vi "RIS.vi"(2 "Run uninterrupted?":bool, 3 "Device Category IN:":string(combo)="Short Strip" caption="Device Category:", 4 "Batch No.:":string, 5 "Wafer Serial No.:":string, 6 "Sensor Serial No.:":string) -> (0 "Done!":bool)   [LabVIEW 2013]
doc: "Performs Ris measurements according to ATLAS ITk Quality Control Specifications."
uses:
  InstrControl/SupplyControl/SupplyControl.lvclass
  general_VIs/globals/QC_RunInformation.vi
  InstrControl/ArduinoControl/ArduinoControl.lvclass
  general_VIs/globals/QC_MeasurementSetup.vi
  <vilib>/Analysis/NI_AALBase.lvlib
  InstrControl/InstrumentSetup.vi
  InstrControl/InstrControl.lvclass
  <vilib>/Analysis/6fits.llb/Curve Fitting Criteria.ctl
  <vilib>/Analysis/NI_AALPro.lvlib
  InstrControl/MultimeterControl/MultimeterControl.lvclass
  InstrControl/Switching/Switching.lvclass
panel:
  out "Ris":dbl[](array[numeric]) caption="Ris [MOhm]"
  out "Volts":dbl[](array[numeric]) caption="Volts [V]"
  out "Current":dbl[](array[numeric]) caption="Current [nA]"
  in  "No. of readouts":i32=5
  out "Risgraph":cluster{dbl[], dbl[]}(graph)
  out "Vigraph":cluster{i32[], dbl[]}[](graph)
  out "Imgraph":cluster{i32[], dbl[]}[](graph)
  out "Initial volts [V]":dbl format="%.1f"
  out "Final volts [V]":dbl=-700.0 format="%.1f"
  out "step [V]":dbl=10.0 format="%.1f"
  out "step interval [s]":u32=10
  out "Temp.":dbl[](array[numeric]) caption="Temp. [°C]" format="%#.2f"
  out "RH":dbl[](array[numeric]) caption="RH [%]" format="%#.2f"
  out "positive ramp?":bool
  out "Tab Control":enum32{"Ris Setup", "Ris Scan"}(tab)
  in  "Voltmeter":string(combo)="Keithley 2410"
  in  "Ris SMU":string(combo)="Keithley 2410"
  in  "Current \nLimit \n[µA]":dbl=1000.0 min=0.0001 format="%.3f"
  in  "Set\ncurrent\nlimit?":bool
  in  "Temperature":enum16{"Read Arduino", "Enter manually"}(ring)
  in  "Ris Supply":string(combo)="Keithley 2410"
  in  "User:":string(combo)="Christoph"
  in  "Configurations":bool
  in  "Manufacturer:":string(combo)="Hamamatsu"
  in  "Quit":bool
  in  "Continue":bool
  in  "abort":bool
  out "Device Category:":string
  out "Batch:":string
  out "Current Volts:":dbl format="%.2f"
  in  "quit (no save)":bool
  in  "Quit & Save":bool
  out "Bias On/Off:":bool
  out "STATUS 1":string
  out "Initiated:":string
  out "Sensor No.:":string
  out "No of steps":u32
  out "Current reading No.":u32
  out "Last reading at:":string
  out "Ris SMU Current [nA]":dbl[][][](array[numeric])
  out "Ris induced Voltage [V]":dbl[][][](array[numeric])
  # "University of\nCambridge"
  # "Strip Sensor QC: inter-strip Resistance"
  # "Ris Scan parameters:"
  # "Last 5 readings:"
  # "n-4"
  # "n-3"
  # "n-2"
  # "n-1"
  # "n"
  # "DUT & Test Description"
  # "Hardware"
  # "DUT & Test Description:"
  # "Current status:"
  # "Rdg No:"
  # "out of"
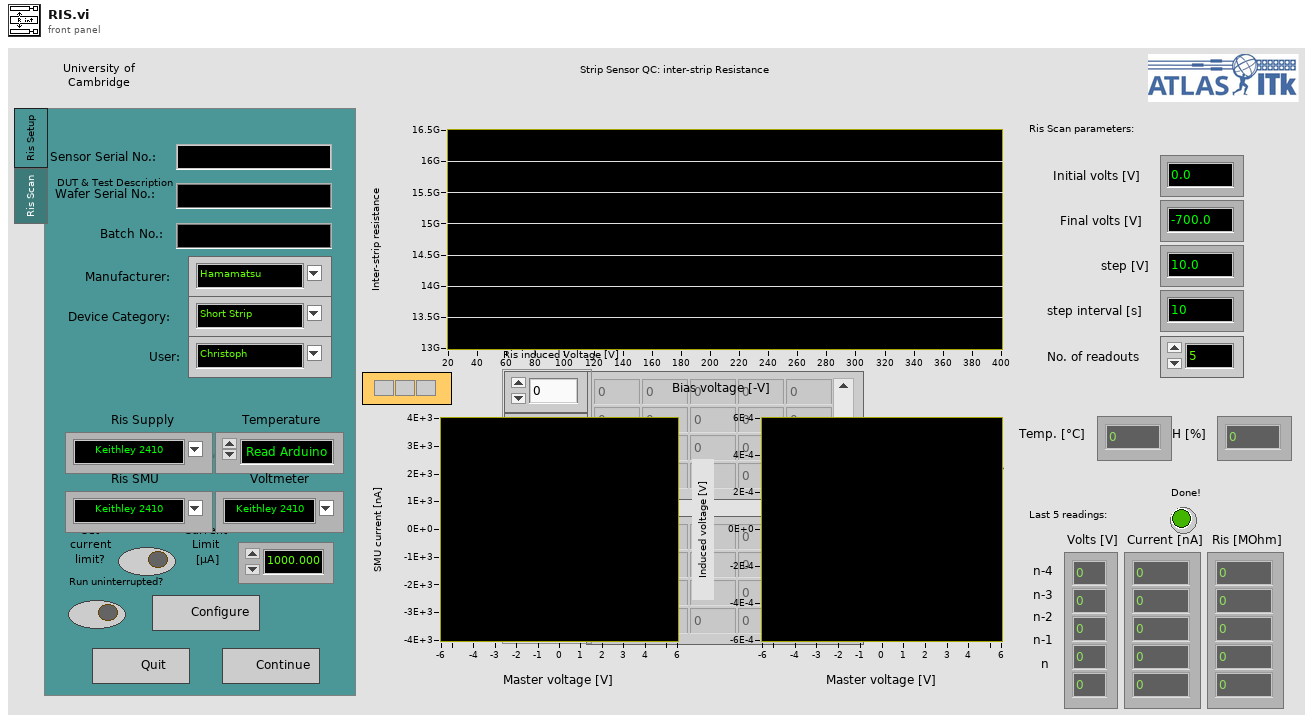
[diagram p1: front panel]
types:
  T1 = enum32{"IV", "CV", "Stability", "Striptest", "Cis", "Ris", "PTP"}
  T2 = enum16{"Supply", "LCR", "Multimeter", "Switching"}
  T3 = enum16{"Reset", "Read Array", "Read Element", "Write Element", "Write Array", "Add Element", "Add Array"}
  T4 = enum16{"Reset", "Ground", "Striptest SMU", "Striptest LCR", "IV", "CV", "Interstrip Cap", "Interstrip Res"}
  T5 = cluster{"Sensor Serial No.:":string, "Wafer:":string, "Batch:":string, "Manufacturer:":string, "Device Category:":string, "Database Serial No.:":string, "Date Initiated:":string, "Time Initiated:":string, "Test":string, "Probeplan used:":string, "End of Run comment:":string, "User:":string, "Vbias SMU":string, "LCR":string, "Test SMU":string, "Test DMM":string}
  T6 = cluster{"Institute":string, "Manufacturers":string[], "Devices":string[], "Serialnumbers Lookup DB":string, "Data directory":string, "Backup & screenshot directory":string, "List of known users":string[], "Measurement switch not used":bool, "Measurement Switch":string, "DUT Switch":string, "Rseries IV [MOhm]":string, "Rshunt IV [MOhm]":string, "Rseries CV [MOhm]":string, "DC blocking Cap [µF]":string, "Rseries LCR [MOhm]":string, "Rseries stability [MOhm]":string, "Rshunt stability [MOhm]":string, "Rseries striptest bias [MOhm]":string, "Rseries strip pinhole [MOhm]":string}
  T7 = cluster{"Bias Supply":refnum<class "SupplyControl.lvclass">, "SMU":refnum<class "SupplyControl.lvclass">, "Multimeter":refnum<class "MultimeterControl.lvclass">, "Arduino":refnum<class "ArduinoControl.lvclass">, "Measurement switch":refnum<class "Switching.lvclass">, "Initial Voltage [V]":dbl, "Final Voltage [V]":dbl, "Step Size [V]":dbl, "Step Interval [s]":i32, "Number Of Steps":u32, "Ramp down steps [V]":dbl, "Ramp down Interval [s]":i32, "Set Current Limit?":bool, "Current Limit [µA]":dbl, "Temperature Readout":enum16{"Read Arduino", "Enter manually"}, "Supply Name":string, "SMU Name":string, "Voltmeter Name":string, "R_is Limit [MOhm]":dbl, "Measurement switch used?":bool, "Matrix X Channels":cluster{"Bias Supply / SMU LO":i32, "Bias Supply / SMU HI":i32, "CV Box LO":i32, "CV Box HI":i32, "CV Box LO IN":i32, "CV Box HI IN":i32, "Volt meter LO":i32, "Volt meter HI":i32, "Mux1 C1":i32, "Mux1 C2":i32, "Mux2 C1":i32, "Mux2 C2":i32}}
  T8 = cluster{"VISA address":refnum<visa-resource-name>, "T sensor":enum16{"SHT", "DS"}, "Arduino":refnum<class "ArduinoControl.lvclass">}
  T9 = typedef "NI_AALPro.lvlib/Curve Fitting Criteria.ctl" = u16
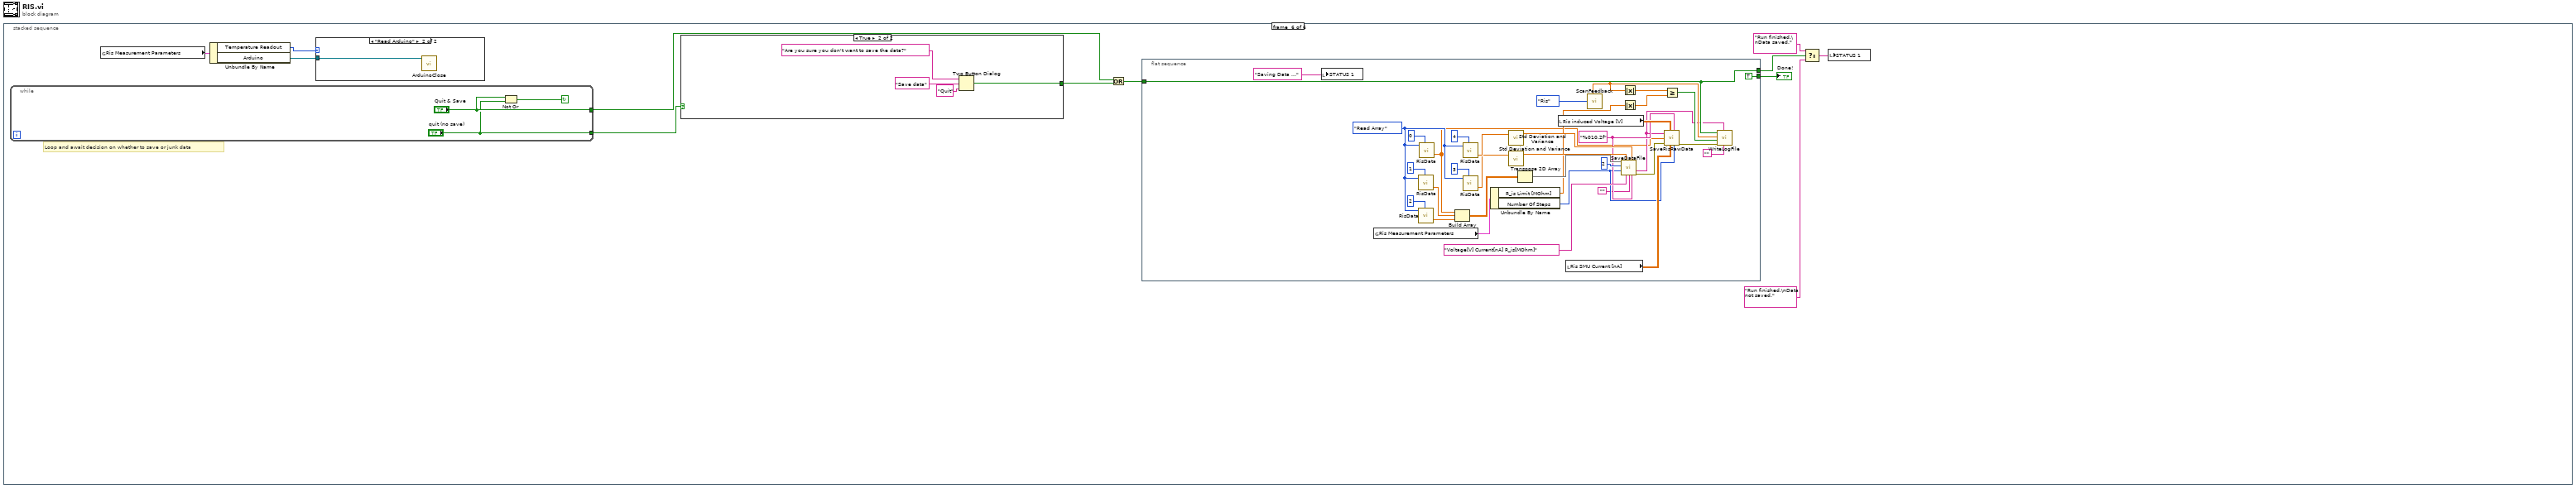
[diagram p0: block diagram]
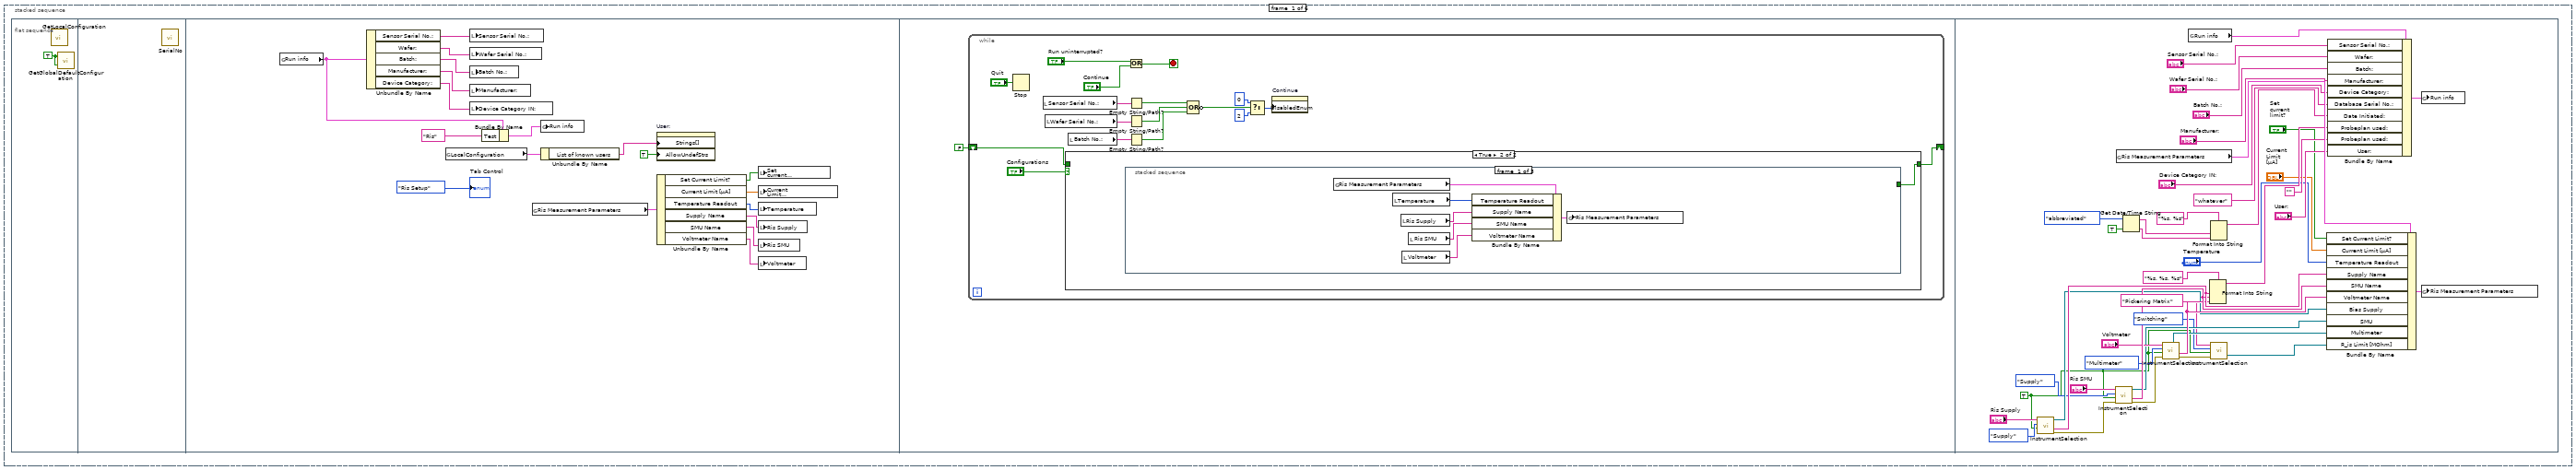
[diagram p2: hidden frame]
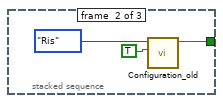
[diagram p4: hidden frame]
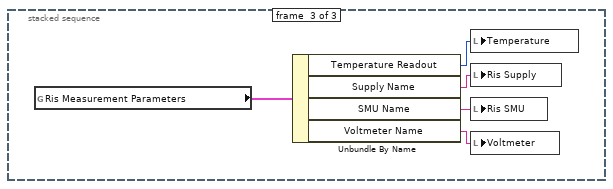
[diagram p5: hidden frame]
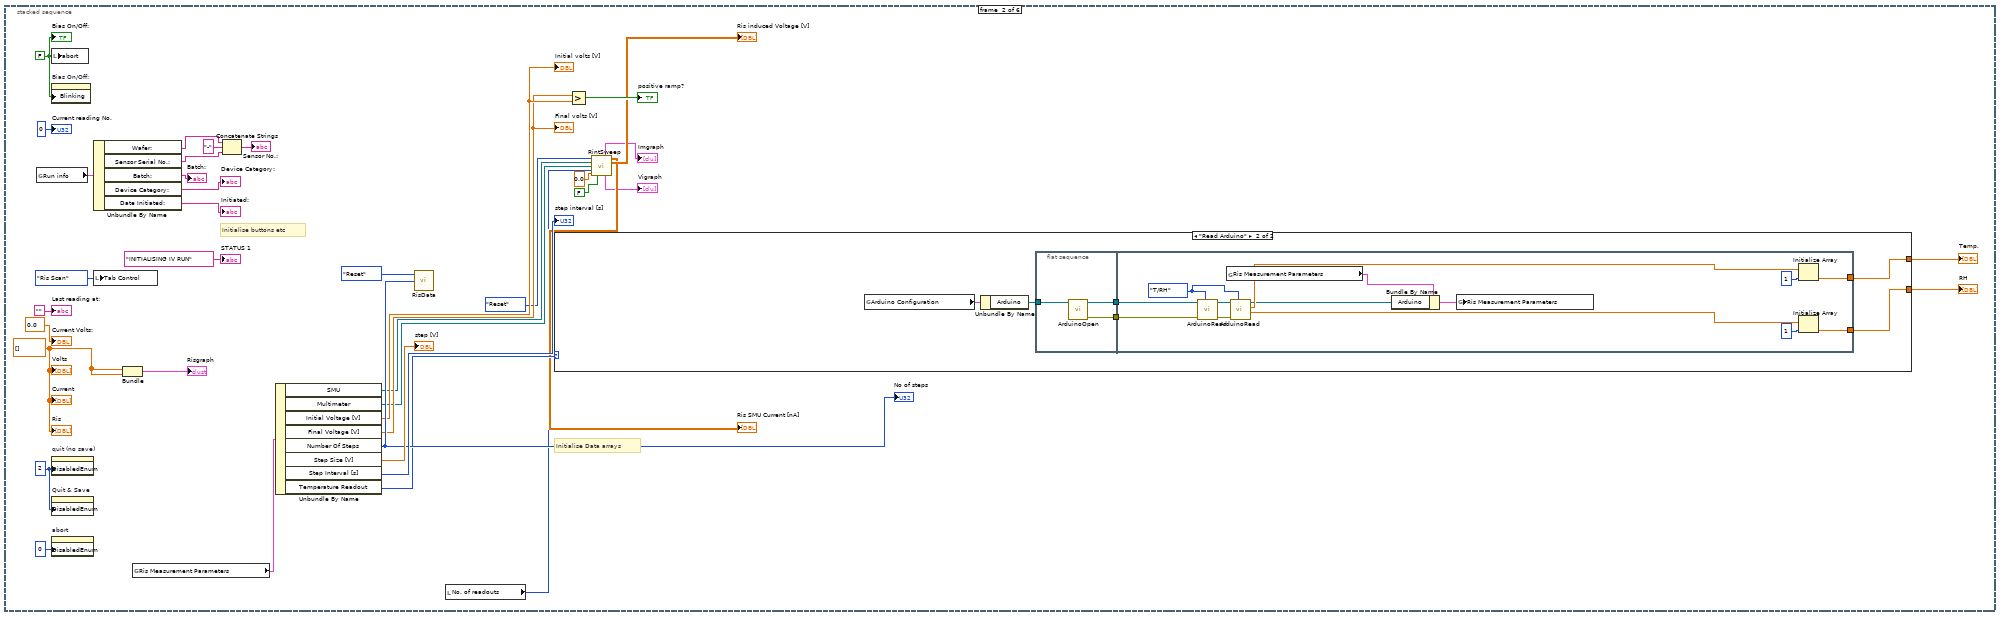
[diagram p6: hidden frame]
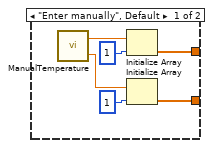
[diagram p7: hidden frame]
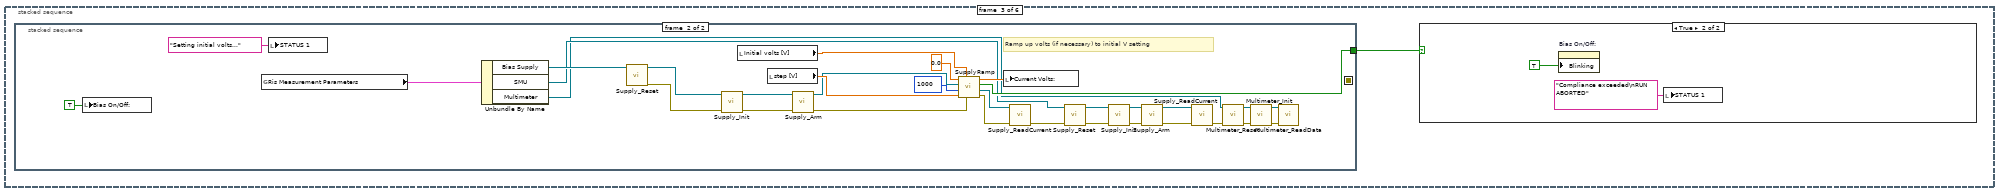
[diagram p8: hidden frame]
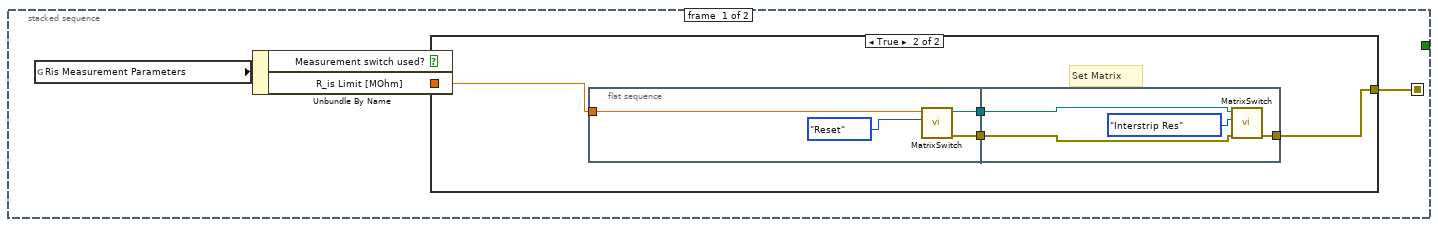
[diagram p9: hidden frame]
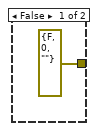
[diagram p10: hidden frame]
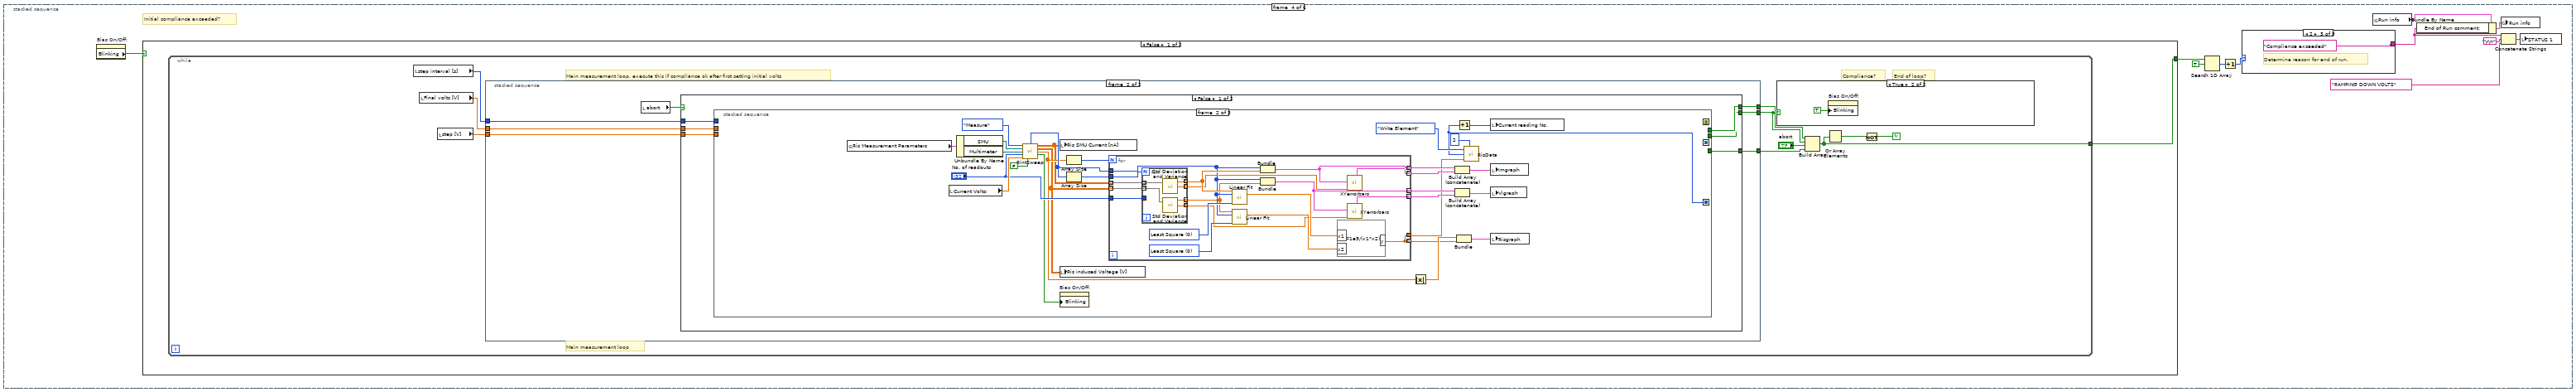
[diagram p12: hidden frame]
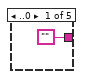
[diagram p13: hidden frame]
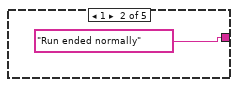
[diagram p14: hidden frame]
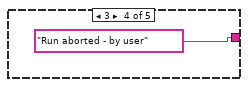
[diagram p15: hidden frame]
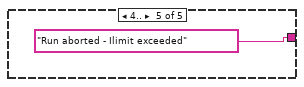
[diagram p16: hidden frame]
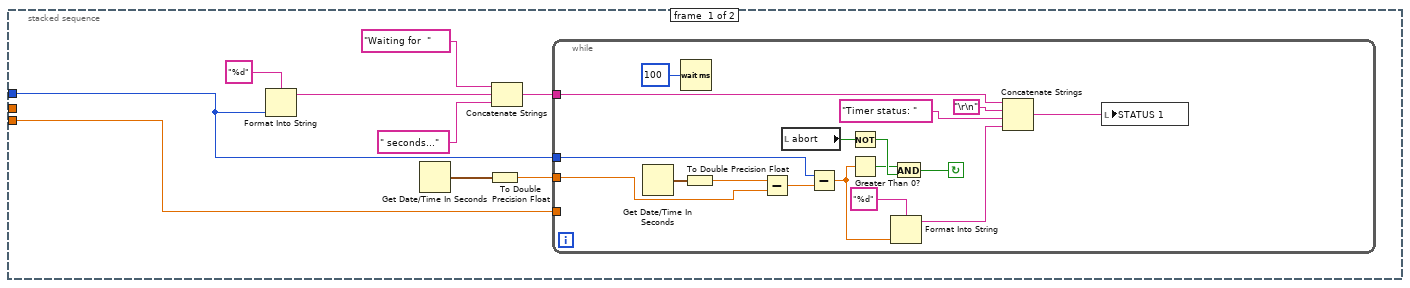
[diagram p17: hidden frame]
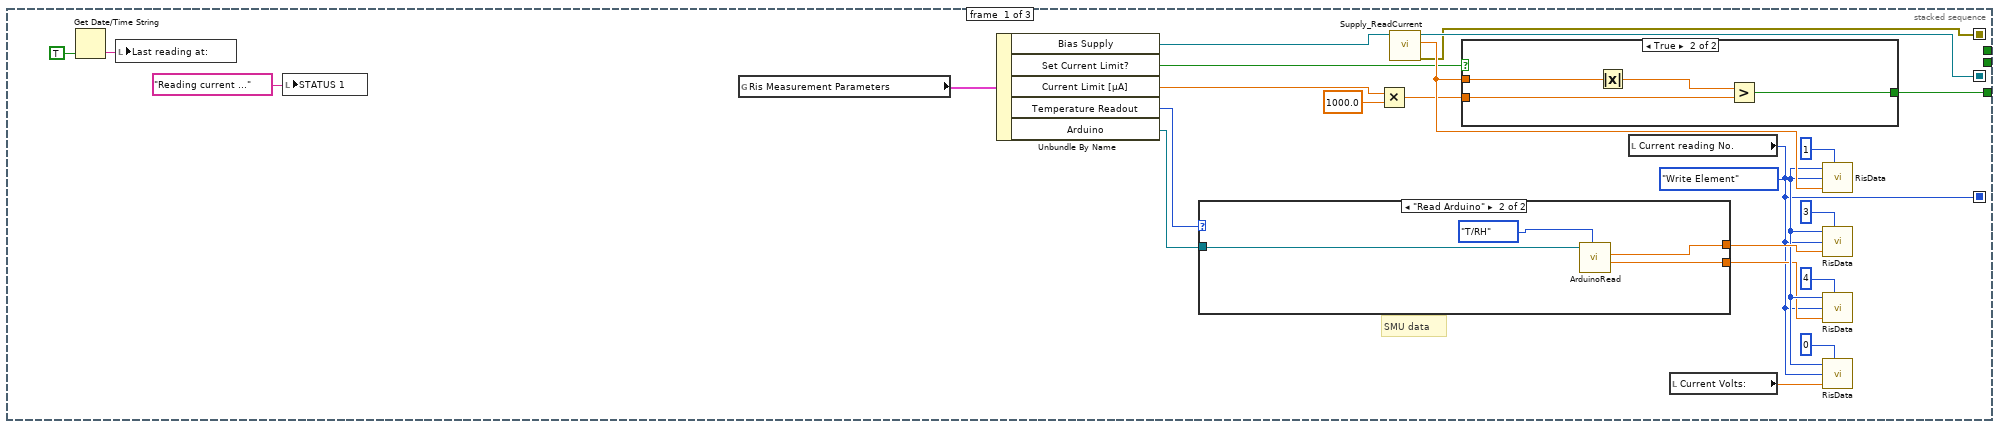
[diagram p18: hidden frame]
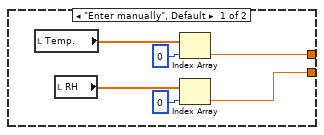
[diagram p19: hidden frame]
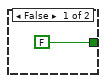
[diagram p20: hidden frame]
diagram:
  n1 = stacked-sequence {
    frame #0 {
      n2 = flat-sequence {
        frame #0 {
          w1 = TRUE
          n3 = call "GetLocalConfiguration.vi"() -> ()  [unwired: 3 in, 1 out]
          n4 = call "GetGlobalDefaultConfiguration.vi"(2:w1, "Read defaults?"=w1) -> ()  [unwired: 2 in]
        }
        frame #1 {
          n5 = call "SerialNo.vi"() -> ()  [unwired: 5 in, 1 out]
        }
        frame #2 {
          n6 = global read "QC_RunInformation.vi" "Run info"() -> (w7:T5)
          n7 = Unbundle By Name(w7) -> ("Sensor Serial No.:"=w3:string, "Wafer:"=w4:string, "Batch:"=w5:string, "Manufacturer:"=w2:string, "Device Category:"=w6:string)
          n8 = global read "QC_RunInformation.vi" "LocalConfiguration"() -> (w15:T6)
          n9 = local write "Sensor Serial No.:"(w3) -> ()
          n10 = local write "Wafer Serial No.:"(w4) -> ()
          n11 = local write "Batch No.:"(w5) -> ()
          n12 = local write "Manufacturer:"(w2) -> ()
          n13 = local write "Device Category IN:"(w6) -> ()
          n14 = Bundle By Name(cluster=w7, "Test"="Ris") -> (w12:T5)
          n15 = global read "QC_MeasurementSetup.vi" "Ris Measurement Parameters"() -> (w18:T7)
          n16 = global write "QC_RunInformation.vi" "Run info"(w12) -> ()
          n17 = Unbundle By Name(w15) -> ("List of known users"=w14:string[])
          n18 = property on="User:" class="CmbBox"("Strings[]"=w14, "AllowUndefStrs"=TRUE) -> ()  [unwired: 2 in, 2 out]
          n19 = Unbundle By Name(w18) -> ("Set Current Limit?"=w17:bool, "Current Limit [µA]"=w16:dbl, "Temperature Readout"=w20:enum16{"Read Arduino", "Enter manually"}, "Supply Name"=w19:string, "SMU Name"=w9:string, "Voltmeter Name"=w8:string)
          n20 = local write "Set\ncurrent\nlimit?"(w17) -> ()
          n21 = local write "Current \nLimit \n[µA]"(w16) -> ()
          n22 = local write "Temperature"(w20) -> ()
          n23 = local write "Ris Supply"(w19) -> ()
          n24 = local write "Ris SMU"(w9) -> ()
          n25 = local write "Voltmeter"(w8) -> ()
          "Tab Control" <- enum32{"Ris Setup", "Ris Scan"}."Ris Setup" ("Tab Control")
        }
        frame #3 {
          n26 = while {
            shift-right: [w26] -> _
            shift-left: FALSE -> [w25]
            stop <- w22 stop-if-true
            n27 = Stop(stop? (T)="Quit") -> ()
            n28 = local read "Sensor Serial No.:"() -> (w37:string)
            n29 = local read "Wafer Serial No.:"() -> (w36:string)
            n30 = case shown="True" "Configurations" {
              tunnel: [w39 w40] -> w26
              tunnel: w25 -> [w39 _]
              frame False {
              }
              frame True {
                n31 = stacked-sequence {
                  tunnel: [_ w47 _] -> w40
                  frame #0 {
                    n32 = global read "QC_MeasurementSetup.vi" "Ris Measurement Parameters"() -> (w46:T7)
                    n33 = local read "Temperature"() -> (w45:enum16{"Read Arduino", "Enter manually"})
                    n34 = local read "Ris Supply"() -> (w44:string)
                    n35 = local read "Voltmeter"() -> (w42:string)
                    n36 = local read "Ris SMU"() -> (w43:string)
                    n37 = Bundle By Name(cluster=w46, "Temperature Readout"=w45, "Supply Name"=w44, "SMU Name"=w43, "Voltmeter Name"=w42) -> (w41:T7)
                    n38 = global write "QC_MeasurementSetup.vi" "Ris Measurement Parameters"(w41) -> ()
                  }
                  frame #1 {
                    n39 = call "Configuration_old.vi"("Open from\nscan VI"=TRUE, "Measurements"=T1."Ris") -> ("configured?"=w47:bool)  [unwired: 9 in]
                  }
                  frame #2 {
                    n40 = global read "QC_MeasurementSetup.vi" "Ris Measurement Parameters"() -> (w54:T7)
                    n41 = Unbundle By Name(w54) -> ("Temperature Readout"=w50:enum16{"Read Arduino", "Enter manually"}, "Supply Name"=w51:string, "SMU Name"=w52:string, "Voltmeter Name"=w53:string)
                    n42 = local write "Temperature"(w50) -> ()
                    n43 = local write "Ris Supply"(w51) -> ()
                    n44 = local write "Ris SMU"(w52) -> ()
                    n45 = local write "Voltmeter"(w53) -> ()
                  }
                }
              }
            }
            n46 = local read "Batch No.:"() -> (w28:string)
            n47 = Or(x="Run uninterrupted?", y="Continue") -> (x .or. y?=w22:bool)
            n48 = Empty String/Path?(string/path=w37) -> (empty?=w34:bool)
            n49 = Empty String/Path?(string/path=w36) -> (empty?=w35:bool)
            n50 = Empty String/Path?(string/path=w28) -> (empty?=w27:bool)
            n51 = Compound Arithmetic op=OR(w34, w35, w27) -> (invert w33:bool)
            n52 = Select(t=0, s=w33, f=2) -> (s? t:f=w30:i32)
            n53 = property on="Continue" class="Bool"("DisabledEnum"=w30) -> ()  [unwired: 2 in, 2 out]
          }
        }
        frame #4 {
          w57 = TRUE
          n54 = call "InstrumentSelection.vi"("Verify GPIB address"=w57, "Instrument type"=T2."Supply", "Instrument name IN"="Ris Supply") -> ("error out"=w64:errorcluster, "Instrument name OUT"=w72:string, "Supply"=w67:refnum<class "SupplyControl.lvclass">)  [unwired: 3 in, 3 out]
          n55 = call "InstrumentSelection.vi"("error in (no error)"=w64, "Verify GPIB address"=w57, "Instrument type"=T2."Supply", "Instrument name IN"="Ris SMU") -> ("error out"=w63:errorcluster, "Instrument name OUT"=w70:string, "Supply"=w66:refnum<class "SupplyControl.lvclass">)  [unwired: 2 in, 3 out]
          n56 = global read "QC_MeasurementSetup.vi" "Ris Measurement Parameters"() -> (w95:T7)
          n57 = Get Date/Time String(date format (0)=enum16{"short", "long", "abbreviated"}."abbreviated", want seconds? (F)=TRUE) -> (date string=w92:string, time string=w91:string)  [unwired: 1 in]
          n58 = call "InstrumentSelection.vi"("error in (no error)"=w63, "Verify GPIB address"=w57, "Instrument type"=T2."Multimeter", "Instrument name IN"="Voltmeter") -> ("error out"=w62:errorcluster, "Instrument name OUT"=w68:string, "Multimeter"=w65:refnum<class "MultimeterControl.lvclass">)  [unwired: 2 in, 3 out]
          n59 = global read "QC_RunInformation.vi" "Run info"() -> (w89:T5)
          n60 = Format Into String(format string="%s, %s, %s", w72, w70, w68) -> (resulting string=w77:string)  [unwired: 2 in, 1 out]
          n61 = Format Into String(format string="%s, %s", w92, w91) -> (resulting string=w87:string)  [unwired: 2 in, 1 out]
          n62 = call "InstrumentSelection.vi"("error in (no error)"=w62, "Verify GPIB address"=w57, "Instrument type"=T2."Switching", "Instrument name IN"="Pickering Matrix") -> ("Switching"=w56:refnum<class "Switching.lvclass">)  [unwired: 2 in, 5 out]
          n63 = Bundle By Name(cluster=w95, "Set Current Limit?"="Set\ncurrent\nlimit?", "Current Limit [µA]"="Current \nLimit \n[µA]", "Temperature Readout"="Temperature", "Supply Name"=w72, "SMU Name"=w70, "Voltmeter Name"=w68, "Bias Supply"=w67, "SMU"=w66, "Multimeter"=w65, "R_is Limit [MOhm]"=w56) -> (w96:T7)
          n64 = Bundle By Name(cluster=w89, "Sensor Serial No.:"="Sensor Serial No.:", "Wafer:"="Wafer Serial No.:", "Batch:"="Batch No.:", "Manufacturer:"="Manufacturer:", "Device Category:"="Device Category IN:", "Database Serial No.:"="whatever", "Date Initiated:"=w87, "Probeplan used:"=w77, "Probeplan used:"="", "User:"="User:") -> (w88:T5)
          n65 = global write "QC_RunInformation.vi" "Run info"(w88) -> ()
          n66 = global write "QC_MeasurementSetup.vi" "Ris Measurement Parameters"(w96) -> ()
        }
      }
    }
    frame #1 {
      w102 = dbl[] []
      w124 = 2
      w123 = FALSE ("Visible")
      # "Initialise buttons etc"
      # "Initialise Data arrays"
      n67 = global read "QC_RunInformation.vi" "Run info"() -> (w134:T5)
      n68 = local write "abort"(w123) -> ()
      n69 = property on="Bias On/Off:" class="Bool (strict)"("Blinking"=w123) -> ()  [unwired: 2 in, 2 out]
      n70 = property on="quit (no save)" class="Bool"("DisabledEnum"=w124) -> ()  [unwired: 2 in, 2 out]
      n71 = property on="Quit & Save" class="Bool"("DisabledEnum"=w124) -> ()  [unwired: 2 in, 2 out]
      n72 = property on="abort" class="Bool (strict)"("DisabledEnum"=0) -> ()  [unwired: 2 in, 2 out]
      n73 = Unbundle By Name(w134) -> ("Wafer:"=w115:string, "Sensor Serial No.:"=w114:string, "Batch:"=→"Batch:":string, "Device Category:"=→"Device Category:":string, "Date Initiated:"=→"Initiated:":string)
      n74 = local write "Tab Control"(enum32{"Ris Setup", "Ris Scan"}."Ris Scan" ("Tab Control")) -> ()
      n75 = Bundle(w102, w102) -> (→"Risgraph":cluster{dbl[], dbl[]})  [unwired: 1 in]
      n76 = global read "QC_MeasurementSetup.vi" "Ris Measurement Parameters"() -> (w117:T7)
      n77 = Concatenate Strings(w115, "-", w114) -> (→"Sensor No.:":string)
      n78 = Unbundle By Name(w117) -> ("SMU"=w98:refnum<class "SupplyControl.lvclass">, "Multimeter"=w97:refnum<class "MultimeterControl.lvclass">, "Initial Voltage [V]"=w122:dbl, "Final Voltage [V]"=w121:dbl, "Number Of Steps"=w130:u32, "Step Size [V]"=→"step [V]":dbl, "Step Interval [s]"=→"step interval [s]":i32, "Temperature Readout"=w125:enum16{"Read Arduino", "Enter manually"})
      "No of steps" <- w130
      "Initial volts [V]" <- w122
      "Final volts [V]" <- w121
      n79 = call "RisData.vi"("Action"=T3."Reset", "Array Size / Index"=w130) -> ()  [unwired: 3 in, 2 out]
      n80 = local read "No. of readouts"() -> (w100:i32)
      n81 = case shown="\"Read Arduino\"" w125 {
        tunnel: [w140 w147] -> w127
        tunnel: [w137 w146] -> w118
        frame "Enter manually", Default {
          n82 = call "ManualTemperature.vi"() -> ("Humidity [%] out"=w136:dbl, "Temperature [°C] out"=w141:dbl)
          n83 = Initialize Array(w141, 1) -> (w140:dbl[])
          n84 = Initialize Array(w136, 1) -> (w137:dbl[])
        }
        frame "Read Arduino" {
          n85 = global read "InstrumentSetup.vi" "Arduino Configuration"() -> (w143:T8)
          n86 = Unbundle By Name(w143) -> ("Arduino"=w142:refnum<class "ArduinoControl.lvclass">)
          n87 = flat-sequence {
            tunnel: [w148] -> w145
            tunnel: [w150] -> w144
            tunnel: w142 -> [w149]
            tunnel: [w164] -> w147
            tunnel: [w161] -> w146
            tunnel: w145 -> [w155]
            tunnel: w144 -> [w154]
            frame #0 {
              n88 = call "ArduinoOpen.vi"("ArduinoControl in"=w149) -> ("error out"=w150:errorcluster, "ArduinoControl out"=w148:refnum<class "ArduinoControl.lvclass">)  [unwired: 9 in]
            }
            frame #1 {
              w151 = enum16{"T/RH", "Interlock", "Edgesense"}."T/RH" ("Arduino function")
              n89 = call "ArduinoRead.vi"("Arduino function"=w151, "error in (no error)"=w154, "ArduinoControl in"=w155) -> ("error out"=w153:errorcluster, "ArduinoControl out"=w152:refnum<class "ArduinoControl.lvclass">)  [unwired: 3 in, 4 out]
              n90 = global read "QC_MeasurementSetup.vi" "Ris Measurement Parameters"() -> (w157:T7)
              n91 = call "ArduinoRead.vi"("Arduino function"=w151, "error in (no error)"=w153, "ArduinoControl in"=w152) -> ("rel. Humidity [%]"=w159:dbl, "Temperature [°C]"=w160:dbl, "ArduinoControl out"=w158:refnum<class "ArduinoControl.lvclass">)  [unwired: 3 in, 3 out]
              n92 = Bundle By Name(cluster=w157, "Arduino"=w158) -> (w156:T7)
              n93 = global write "QC_MeasurementSetup.vi" "Ris Measurement Parameters"(w156) -> ()
              n94 = Initialize Array(w160, 1) -> (w164:dbl[])
              n95 = Initialize Array(w159, 1) -> (w161:dbl[])
            }
          }
        }
      }
      "Temp." <- w127
      "RH" <- w118
      n96 = Greater?(x=w121, y=w122) -> (0:→"positive ramp?":bool)
      n97 = call "RintSweep.vi"("Action"=enum16{"Reset", "Measure"}."Reset", "MasterVoltage Supply in"=w98, "VoltmeterControl in"=w97, "No. of readouts"=w100, "Bias [V]"=0.0, "Simulated data?"=FALSE) -> ("Igraph"=→"Imgraph":cluster{i32[], dbl[]}[], "Applied Current [nA]"=→"Ris SMU Current [nA]":dbl[][][], "Induced Voltage [V]"=→"Ris induced Voltage [V]":dbl[][][], "ViGraph"=→"Vigraph":cluster{i32[], dbl[]}[])  [unwired: 2 in, 4 out]
      "STATUS 1" <- "INITIALISING IV RUN"
      "Bias On/Off:" <- w123
      "Last reading at:" <- ""
      "Current reading No." <- u32 0 ("Current reading No.")
      "Current Volts:" <- 0.0 ("Current Volts:")
      "Current" <- w102
      "Volts" <- w102
      "Ris" <- w102
    }
    frame #2 {
      n98 = stacked-sequence {
        seq-local: [w167 _] -> [_ _]
        tunnel: [_ w197] -> w165
        frame #0 {
          n99 = global read "QC_MeasurementSetup.vi" "Ris Measurement Parameters"() -> (w166:T7)
          n100 = Unbundle By Name(w166) -> ("Measurement switch used?"=w169:bool, "R_is Limit [MOhm]"=w168:dbl)
          n101 = case shown="True" w169 {
            tunnel: w168 -> [_ w171]
            tunnel: [errorcluster {"status"=FALSE, "code"=0, "source"=""} ("error constant") w172] -> w167
            frame False {
            }
            frame True {
              # "Set Matrix"
              n102 = flat-sequence {
                tunnel: [w178] -> w174
                tunnel: [w177] -> w173
                tunnel: w171 -> [w175]
                tunnel: w174 -> [w182]
                tunnel: w173 -> [w181]
                tunnel: [w180] -> w172
                frame #0 {
                  n103 = call-dynamic "MatrixSwitch.vi"("Action"=T4."Reset", "Switching in"=w175) -> ("error out"=w178:errorcluster, "Switching out"=w177:refnum<class "Switching.lvclass">)  [unwired: 7 in, 1 out]
                }
                frame #1 {
                  n104 = call-dynamic "MatrixSwitch.vi"("error in (no error)"=w182, "Action"=T4."Interstrip Res", "Switching in"=w181) -> ("error out"=w180:errorcluster)  [unwired: 6 in, 2 out]
                }
              }
            }
          }
        }
        frame #1 {
          # "Ramp up volts (if necessary) to initial V setting"
          n105 = local write "Bias On/Off:"(TRUE ("Compliance?")) -> ()
          n106 = global read "QC_MeasurementSetup.vi" "Ris Measurement Parameters"() -> (w210:T7)
          n107 = local write "STATUS 1"("Setting initial volts..." ("STATUS 1")) -> ()
          n108 = Unbundle By Name(w210) -> ("Bias Supply"=w207:refnum<class "SupplyControl.lvclass">, "SMU"=w189:refnum<class "SupplyControl.lvclass">, "Multimeter"=w184:refnum<class "MultimeterControl.lvclass">)
          n109 = call-dynamic "Supply_Reset.vi"("SupplyControl in"=w207) -> ("error out"=w212:errorcluster, "SupplyControl out"=w214:refnum<class "SupplyControl.lvclass">)  [unwired: 9 in]
          n110 = call-dynamic "Supply_Init.vi"("error in (no error)"=w212, "SupplyControl in"=w214) -> ("error out"=w211:errorcluster, "SupplyControl out"=w213:refnum<class "SupplyControl.lvclass">)  [unwired: 8 in]
          n111 = local read "Initial volts [V]"() -> (w200:dbl)
          n112 = local read "step [V]"() -> (w201:dbl)
          n113 = call-dynamic "Supply_Arm.vi"("error in (no error)"=w211, "SupplyControl in"=w213) -> ("error out"=w199:errorcluster, "SupplyControl out"=w198:refnum<class "SupplyControl.lvclass">)  [unwired: 8 in]
          n114 = call "SupplyRamp.vi"("error in"=w199, "Requested Voltage"=w200, "Step Size"=w201, "Step Delay"=1000, "Supply IN"=w198, "Starting Voltage"=0.0) -> ("error out"=w205:errorcluster, "Supply OUT"=w206:refnum<class "SupplyControl.lvclass">, "Compliance exceeded"=w197:bool, "Current Voltage"=w204:dbl)  [unwired: 2 in]
          n115 = local write "Current Volts:"(w204) -> ()
          n116 = call-dynamic "Supply_ReadCurrent.vi"("error in (no error)"=w205, "SupplyControl in"=w206) -> ("error out"=w190:errorcluster)  [unwired: 7 in, 2 out]
          n117 = call-dynamic "Supply_Reset.vi"("error in (no error)"=w190, "SupplyControl in"=w189) -> ("error out"=w194:errorcluster, "SupplyControl out"=w196:refnum<class "SupplyControl.lvclass">)  [unwired: 8 in]
          n118 = call-dynamic "Supply_Init.vi"("error in (no error)"=w194, "SupplyControl in"=w196) -> ("error out"=w193:errorcluster, "SupplyControl out"=w195:refnum<class "SupplyControl.lvclass">)  [unwired: 8 in]
          n119 = call-dynamic "Supply_Arm.vi"("error in (no error)"=w193, "SupplyControl in"=w195) -> ("error out"=w192:errorcluster, "SupplyControl out"=w191:refnum<class "SupplyControl.lvclass">)  [unwired: 8 in]
          n120 = call-dynamic "Supply_ReadCurrent.vi"("error in (no error)"=w192, "SupplyControl in"=w191) -> ("error out"=w183:errorcluster)  [unwired: 7 in, 2 out]
          n121 = call-dynamic "Multimeter_Reset.vi"("error in (no error)"=w183, "MultimeterControl in"=w184) -> ("error out"=w185:errorcluster, "MultimeterControl out"=w186:refnum<class "MultimeterControl.lvclass">)  [unwired: 8 in]
          n122 = call-dynamic "Multimeter_Init.vi"("error in (no error)"=w185, "MultimeterControl in"=w186) -> ("error out"=w188:errorcluster, "MultimeterControl out"=w187:refnum<class "MultimeterControl.lvclass">)  [unwired: 8 in]
          n123 = call-dynamic "Multimeter_ReadData.vi"("error in (no error)"=w188, "MultimeterControl in"=w187) -> ()  [unwired: 7 in, 3 out]
        }
      }
      n124 = case shown="True" w165 {
        frame False {
        }
        frame True {
          n125 = property on="Bias On/Off:" class="Bool (strict)"("Blinking"=TRUE) -> ()  [unwired: 2 in, 2 out]
          n126 = local write "STATUS 1"("Compliance exceeded\nRUN ABORTED") -> ()
        }
      }
    }
    frame #3 {
      # "Initial compliance exceeded?"
      n127 = property on="Bias On/Off:" class="Bool (strict)"() -> ("Blinking"=w227:bool)  [unwired: 2 in, 2 out]
      n128 = case shown="False" w227 {
        tunnel: [w233 w415] -> w226
        frame False {
          n129 = while {
            tunnel: [w241] -> w233
            stop <- w242 continue-if-true
            # "Main measurement loop"
            # "End of loop?"
            # "Compliance?"
            # "Main measurement loop. execute this if compliance ok after first setting initial volts"
            n130 = local read "step interval [s]"() -> (w238:u32)
            n131 = local read "Final volts [V]"() -> (w239:dbl)
            n132 = local read "step [V]"() -> (w240:dbl)
            n133 = stacked-sequence {
              tunnel: w240 -> [w252 w276]
              tunnel: [_ w275] -> w235
              tunnel: w239 -> [_ w274]
              tunnel: w238 -> [w244 w273]
              tunnel: [_ w272] -> w237
              tunnel: [_ w270] -> w236
              frame #0 {
                n134 = Format Into String(format string="%d", w244) -> (resulting string=w249:string)  [unwired: 2 in, 1 out]
                n135 = Get Date/Time In Seconds() -> (seconds since 1Jan1904=w246:timestamp)
                n136 = To Double Precision Float(number=w246) -> (double precision float=w247:dbl)
                n137 = Concatenate Strings("Waiting for  ", w249, " seconds...") -> (w245:string)
                n138 = while {
                  tunnel: w252 -> [_]
                  tunnel: w245 -> [w257]
                  tunnel: w244 -> [w263]
                  tunnel: w247 -> [w264]
                  stop <- w265 continue-if-true
                  n139 = Get Date/Time In Seconds() -> (seconds since 1Jan1904=w256:timestamp)
                  n140 = Wait (ms)(milliseconds to wait=u32 100) -> ()  [unwired: 1 out]
                  n141 = To Double Precision Float(number=w256) -> (double precision float=w269:dbl)
                  n142 = Subtract(x=w269, y=w264) -> (x-y=w254:dbl)
                  n143 = local read "abort"() -> (w262:bool)
                  n144 = Subtract(x=w263, y=w254) -> (x-y=w253:dbl)
                  n145 = Not(x=w262) -> (.not. x?=w268:bool)
                  n146 = Greater Than 0?(x=w253) -> (x > 0?=w255:bool)
                  n147 = Format Into String(format string="%d", w253) -> (resulting string=w267:string)  [unwired: 2 in, 1 out]
                  n148 = And(x=w255, y=w268) -> (x .and. y?=w265:bool)
                  n149 = Concatenate Strings(w257, "\r\n", "Timer status: ", w267) -> (w261:string)
                  n150 = local write "STATUS 1"(w261) -> ()
                }
              }
              frame #1 {
                n151 = local read "abort"() -> (w271:bool)
                n152 = case shown="False" w271 {
                  tunnel: [w282 w412] -> w272
                  tunnel: w273 -> [w281 _]
                  tunnel: w274 -> [w280 _]
                  tunnel: [w278 w412] -> w275
                  tunnel: w276 -> [w279 _]
                  tunnel: [w277 w412] -> w270
                  frame False {
                    n153 = stacked-sequence {
                      seq-local: [w283 _ _] -> [_ w323 _]
                      seq-local: [w293 _ _] -> [_ _ w381]
                      seq-local: [w292 _ _] -> [_ _ w382]
                      tunnel: w279 -> [_ _ w387]
                      tunnel: w280 -> [_ _ w378]
                      tunnel: [_ _ w385] -> w282
                      tunnel: [_ _ w384] -> w278
                      tunnel: w281 -> [_ _ _]
                      tunnel: [w300 _ _] -> w277
                      frame #0 {
                        w295 = T3."Write Element" ("Action")
                        # "SMU data"
                        n154 = Get Date/Time String(want seconds? (F)=TRUE) -> (time string=w297:string)  [unwired: 2 in, 1 out]
                        n155 = local write "Last reading at:"(w297) -> ()
                        n156 = local write "STATUS 1"("Reading current ..." ("status")) -> ()
                        n157 = global read "QC_MeasurementSetup.vi" "Ris Measurement Parameters"() -> (w291:T7)
                        n158 = Unbundle By Name(w291) -> ("Bias Supply"=w285:refnum<class "SupplyControl.lvclass">, "Set Current Limit?"=w290:bool, "Current Limit [µA]"=w287:dbl, "Temperature Readout"=w289:enum16{"Read Arduino", "Enter manually"}, "Arduino"=w284:refnum<class "ArduinoControl.lvclass">)
                        n159 = case shown="\"Read Arduino\"" w289 {
                          tunnel: [w310 w316] -> w298
                          tunnel: [w307 w315] -> w294
                          tunnel: w284 -> [_ w314]
                          frame "Enter manually", Default {
                            n160 = local read "Temp."() -> (w312:dbl[])
                            n161 = local read "RH"() -> (w308:dbl[])
                            n162 = Index Array(array=w312, index=0) -> (element=w310:dbl)
                            n163 = Index Array(array=w308, index=0) -> (element=w307:dbl)
                          }
                          frame "Read Arduino" {
                            n164 = call "ArduinoRead.vi"("Arduino function"=enum16{"T/RH", "Interlock", "Edgesense"}."T/RH", "ArduinoControl in"=w314) -> ("rel. Humidity [%]"=w315:dbl, "Temperature [°C]"=w316:dbl)  [unwired: 4 in, 4 out]
                          }
                        }
                        n165 = Multiply(x=w287, y=1000.0) -> (x*y=w286:dbl)
                        n166 = call-dynamic "Supply_ReadCurrent.vi"("SupplyControl in"=w285) -> ("error out"=w292:errorcluster, "Current in nA"=w301:dbl, "SupplyControl out"=w293:refnum<class "SupplyControl.lvclass">)  [unwired: 8 in]
                        n167 = case shown="True" w290 {
                          tunnel: w301 -> [_ w321]
                          tunnel: w286 -> [_ w319]
                          tunnel: [FALSE w318] -> w300
                          frame False {
                          }
                          frame True {
                            n168 = Absolute Value(x=w321) -> (abs(x)=w320:dbl)
                            n169 = Greater?(x=w320, y=w319) -> (0:w318:bool)
                          }
                        }
                        n170 = local read "Current reading No."() -> (w283:u32)
                        n171 = local read "Current Volts:"() -> (w302:dbl)
                        n172 = call "RisData.vi"("Action"=w295, "Array No."=u32 1, "Array Size / Index"=w283, "Data IN"=w301) -> ()  [unwired: 1 in, 2 out]
                        n173 = call "RisData.vi"("Action"=w295, "Array No."=u32 3, "Array Size / Index"=w283, "Data IN"=w298) -> ()  [unwired: 1 in, 2 out]
                        n174 = call "RisData.vi"("Action"=w295, "Array No."=u32 4, "Array Size / Index"=w283, "Data IN"=w294) -> ()  [unwired: 1 in, 2 out]
                        n175 = call "RisData.vi"("Action"=w295, "Array No."=0, "Array Size / Index"=w283, "Data IN"=w302) -> ()  [unwired: 1 in, 2 out]
                      }
                      frame #1 {
                        n176 = global read "QC_MeasurementSetup.vi" "Ris Measurement Parameters"() -> (w342:T7)
                        n177 = local read "Current Volts:"() -> (w345:dbl)
                        n178 = Unbundle By Name(w342) -> ("SMU"=w341:refnum<class "SupplyControl.lvclass">, "Multimeter"=w340:refnum<class "MultimeterControl.lvclass">)
                        n179 = call "RintSweep.vi"("Action"=enum16{"Reset", "Measure"}."Measure", "MasterVoltage Supply in"=w341, "VoltmeterControl in"=w340, "No. of readouts"="No. of readouts", "Bias [V]"=w345, "Simulated data?"=FALSE) -> ("Sweep"=w349:i32[], "Applied Current [nA]"=w329:dbl[][][], "Induced Voltage [V]"=w330:dbl[][][], "Voltages OUT"=w332:dbl[], "Compliance exceeded?"=w339:bool)  [unwired: 2 in, 3 out]
                        n180 = local write "Ris SMU Current [nA]"(w329) -> ()
                        n181 = local write "Ris induced Voltage [V]"(w330) -> ()
                        n182 = property on="Bias On/Off:" class="Bool (strict)"("Blinking"=w339) -> ()  [unwired: 2 in, 2 out]
                        n183 = Array Size(array=w332) -> (size(s)=w347:i32)
                        n184 = Array Size(array=w349) -> (size(s)=w348:i32)
                        n185 = for {
                          N: w347 -> [_]
                          tunnel: "No. of readouts" -> [w367]
                          tunnel: w348 -> [w366]
                          tunnel: w329 -> [w365] mode=indexing
                          tunnel: w330 -> [w364] mode=indexing
                          tunnel: w349 -> [w360]
                          tunnel: [w355] -> w338 mode=indexing
                          tunnel: [w354] -> w335 mode=indexing
                          tunnel: [w356] -> w328 mode=indexing
                          tunnel: [w356] -> w324
                          tunnel: [w351] -> w337 mode=indexing
                          tunnel: [w350] -> w334 mode=indexing
                          w363 = T9 0 items=["Least Square", "Least Absolute Residual", "Bisquare"] ("method")
                          w362 = T9 0 items=["Least Square", "Least Absolute Residual", "Bisquare"] ("method")
                          n186 = for {
                            N: w366 -> [_]
                            tunnel: w367 -> [_]
                            tunnel: w365 -> [w373] mode=indexing
                            tunnel: w364 -> [w372] mode=indexing
                            tunnel: [w371] -> w361 mode=indexing
                            tunnel: [w370] -> w359 mode=indexing
                            tunnel: [w369] -> w352 mode=indexing
                            tunnel: [w368] -> w353 mode=indexing
                            n187 = call <vilib>:"Std Deviation and Variance.vi"("X"=w373) -> ("mean"=w371:dbl, "standard deviation"=w369:dbl)  [unwired: 1 in, 1 out]
                            n188 = call <vilib>:"Std Deviation and Variance.vi"("X"=w372) -> ("mean"=w370:dbl, "standard deviation"=w368:dbl)  [unwired: 1 in, 1 out]
                          }
                          n189 = call <vilib>:"Linear Fit.vi"("Y"=w361, "X"=w360, "method"=w363) -> ("slope"=w357:dbl)  [unwired: 8 in, 4 out]
                          n190 = call <vilib>:"Linear Fit.vi"("Y"=w359, "X"=w360, "method"=w362) -> ("slope"=w358:dbl)  [unwired: 8 in, 4 out]
                          n191 = Bundle("Sweep"=w360, w361) -> (w355:cluster{"Sweep":i32[], dbl[]})  [unwired: 1 in]
                          n192 = Bundle("Sweep"=w360, w359) -> (w354:cluster{"Sweep":i32[], dbl[]})  [unwired: 1 in]
                          n193 = formula code="y=1e9/(x1*x2);"("x1"=w357, "x2"=w358) -> ("y"=w356:dbl)
                          n194 = call "XYerrorbars.vi"("XY plot"=w355, "Yerror"=w352) -> ("Y error bars"=w351:cluster{dbl[], dbl[]})  [unwired: 6 in, 2 out]
                          n195 = call "XYerrorbars.vi"("XY plot"=w354, "Yerror"=w353) -> ("Y error bars"=w350:cluster{dbl[], dbl[]})  [unwired: 6 in, 2 out]
                        }
                        n196 = Absolute Value(x=w332) -> (abs(x)=w331:dbl[])
                        n197 = Build Array (concatenate)(w338, w337) -> (w336:cluster{"Sweep":dbl[], dbl[]}[])
                        n198 = Build Array (concatenate)(w335, w334) -> (w333:cluster{"Sweep":dbl[], dbl[]}[])
                        n199 = Bundle(w331, w328) -> (w327:cluster{dbl[], dbl[]})  [unwired: 1 in]
                        n200 = Increment(x=w323) -> (x+1=w322:u32)
                        n201 = call "RisData.vi"("Action"=T3."Write Element", "Array No."=2, "Array Size / Index"=w323, "Data IN"=w324) -> ()  [unwired: 1 in, 2 out]
                        n202 = local write "Current reading No."(w322) -> ()
                        n203 = local write "Imgraph"(w336) -> ()
                        n204 = local write "Vigraph"(w333) -> ()
                        n205 = local write "Risgraph"(w327) -> ()
                      }
                      frame #2 {
                        # "Increment volts and check for end of loop"
                        n206 = local read "positive ramp?"() -> (w383:bool)
                        n207 = local read "Current Volts:"() -> (w379:dbl)
                        n208 = case shown="True" w383 {
                          tunnel: w378 -> [w390 w394]
                          tunnel: w387 -> [w391 w397]
                          tunnel: [w389 w396] -> w374
                          tunnel: [w388 w393] -> w386
                          tunnel: w379 -> [w392 w395]
                          frame False {
                            n209 = Subtract(x=w392, y=w391) -> (x-y=w388:dbl)
                            n210 = Greater Or Equal?(x=w388, y=w390) -> (x >= y?=w389:bool)
                          }
                          frame True {
                            n211 = Add(x=w395, y=w397) -> (x+y=w393:dbl)
                            n212 = Less Or Equal?(x=w393, y=w394) -> (x <= y?=w396:bool)
                          }
                        }
                        n213 = Quotient & Remainder(x=w379, y=w378) -> (x-y*floor(x/y)=w380:dbl, floor(x/y)=w377:dbl)
                        n214 = Not Equal To 0?(x=w380) -> (x != 0?=w375:bool)
                        n215 = Equal To 0?(x=w377) -> (x = 0?=w376:bool)
                        n216 = Or(x=w375, y=w376) -> ()  [unwired: 1 out]
                        n217 = case shown="True" w374 {
                          tunnel: w386 -> [_ w408]
                          tunnel: [TRUE FALSE] -> w385
                          tunnel: [FALSE w409] -> w384
                          tunnel: w379 -> [_ w406]
                          tunnel: w382 -> [_ w405]
                          tunnel: w381 -> [_ w404]
                          frame False {
                          }
                          frame True {
                            n218 = local read "step [V]"() -> (w402:dbl)
                            n219 = call "SupplyRamp.vi"("error in"=w405, "Requested Voltage"=w408, "Step Size"=w402, "Step Delay"=100, "Supply IN"=w404, "Starting Voltage"=w406) -> ("error out"=w400:errorcluster, "Compliance exceeded"=w409:bool, "Current Voltage"=w403:dbl)  [unwired: 2 in, 1 out]
                            n220 = local write "STATUS 1"("Incrementing volts.") -> ()
                            n221 = case shown="No Error" w400 {
                              tunnel: w403 -> [w411 _]
                              frame No Error {
                                n222 = local write "Current Volts:"(w411) -> ()
                              }
                              frame Error {
                              }
                            }
                            n223 = property on="Bias On/Off:" class="Bool (strict)"("Blinking"=w409) -> ()  [unwired: 2 in, 2 out]
                          }
                        }
                      }
                    }
                  }
                  frame True {
                    w412 = FALSE
                  }
                }
              }
            }
            n224 = case shown="True" w235 {
              frame False {
              }
              frame True {
                n225 = property on="Bias On/Off:" class="Bool (strict)"("Blinking"=TRUE) -> ()  [unwired: 2 in, 2 out]
              }
            }
            n226 = Build Array(w237, w235, "abort", w236) -> (w241:bool[])
            n227 = Or Array Elements(Boolean array=w241) -> (logical OR=w243:bool)
            n228 = Not(x=w243) -> (.not. x?=w242:bool)
          }
        }
        frame True {
          w414 = FALSE
          # "compliance was exceeded when first voltage applied."
          # "Flag compliance as reason for end of run"
          n229 = local write "STATUS 1"("Run aborted - compliance exceeded.") -> ()
          n230 = Build Array(w414, TRUE, w414, w414) -> (w415:bool[])
        }
      }
      n231 = Search 1D Array(1D array=w226, element=TRUE) -> (index of element=w224:i32)  [unwired: 1 in]
      n232 = Increment(x=w224) -> (x+1=w223:i32)
      n233 = case shown="2" w223 {
        tunnel: ["" "Run ended normally" "Compliance exceeded" "Run aborted - by user" "Run aborted - Ilimit exceeded"] -> w218
        frame ..0 {
        }
        frame 1 {
        }
        frame 2 {
          # "Determine reason for end of run."
        }
        frame 3 {
        }
        frame 4.. {
        }
      }
      n234 = global read "QC_RunInformation.vi" "Run info"() -> (w222:T5)
      n235 = Bundle By Name(cluster=w222, "End of Run comment:"=w218) -> (w217:T5)
      n236 = global write "QC_RunInformation.vi" "Run info"(w217) -> ()
      n237 = Concatenate Strings(w218, "\r\n", "RAMPING DOWN VOLTS") -> (w221:string)
      n238 = local write "STATUS 1"(w221) -> ()
    }
    frame #4 {
      n239 = stacked-sequence {
        frame #0 {
          # "Tie up loose ends. Set volts to zero and switch to standby"
          # "Ramp down volts now"
          n240 = global read "QC_MeasurementSetup.vi" "Ris Measurement Parameters"() -> (w423:T7)
          n241 = Unbundle By Name(w423) -> ("SMU"=w419:refnum<class "SupplyControl.lvclass">, "Bias Supply"=w420:refnum<class "SupplyControl.lvclass">, "Ramp down steps [V]"=w422:dbl, "Ramp down Interval [s]"=w421:i32, "Multimeter"=w433:refnum<class "MultimeterControl.lvclass">, "R_is Limit [MOhm]"=w434:dbl, "Measurement switch used?"=w435:bool)
          n242 = Multiply(x=w421, y=1000) -> (x*y=w425:i32)
          n243 = local read "Current Volts:"() -> (w428:dbl)
          n244 = call-dynamic "Supply_Stby.vi"("SupplyControl in"=w419) -> ("error out"=w418:errorcluster)  [unwired: 9 in, 1 out]
          n245 = call "SupplyRamp.vi"("error in"=w418, "Requested Voltage"=0.0, "Step Size"=w422, "Step Delay"=w425, "Supply IN"=w420, "Starting Voltage"=w428) -> ("error out"=w430:errorcluster, "Supply OUT"=w429:refnum<class "SupplyControl.lvclass">, "Current Voltage"=w426:dbl)  [unwired: 2 in, 1 out]
          n246 = local write "Current Volts:"(w426) -> ()
          n247 = call-dynamic "Supply_Stby.vi"("error in (no error)"=w430, "SupplyControl in"=w429) -> ("error out"=w431:errorcluster)  [unwired: 8 in, 1 out]
          n248 = call-dynamic "Multimeter_Reset.vi"("error in (no error)"=w431, "MultimeterControl in"=w433) -> ("error out"=w432:errorcluster)  [unwired: 8 in, 1 out]
          n249 = case shown="True" w435 {
            tunnel: w434 -> [_ w438]
            tunnel: w432 -> [_ w437]
            frame False {
            }
            frame True {
              n250 = call-dynamic "MatrixSwitch.vi"("error in (no error)"=w437, "Action"=T4."Reset", "Switching in"=w438) -> ()  [unwired: 6 in, 3 out]
            }
          }
        }
        frame #1 {
          w443 = 0
          n251 = local write "Bias On/Off:"(FALSE ("Visible")) -> ()
          n252 = local write "Current Volts:"(0.0 ("Current Volts:")) -> ()
          n253 = property on="Quit & Save" class="Bool"("DisabledEnum"=w443) -> ()  [unwired: 2 in, 2 out]
          n254 = property on="quit (no save)" class="Bool"("DisabledEnum"=w443) -> ()  [unwired: 2 in, 2 out]
          n255 = property on="abort" class="Bool (strict)"("DisabledEnum"=2) -> ()  [unwired: 2 in, 2 out]
          n256 = local write "STATUS 1"("Run finished. \nSave data?" ("STATUS 1")) -> ()
        }
        frame #2 {
          n257 = Current VI's Path() -> (path=w445:path)
          n258 = call "SaveJPEG.vi"("Test"="Ris", "File Path Control"=w445) -> ()  [unwired: 1 in, 2 out]
        }
      }
    }
    frame #5 {
      # "Loop and await decision on whether to save or junk data"
      n259 = while {
        tunnel: ["Quit & Save"] -> w456
        tunnel: ["quit (no save)"] -> w455
        stop <- w496 continue-if-true
        n260 = Not Or(1:"quit (no save)", 2:"Quit & Save") -> (0:w496:bool)
      }
      n261 = global read "QC_MeasurementSetup.vi" "Ris Measurement Parameters"() -> (w454:T7)
      n262 = Unbundle By Name(w454) -> ("Temperature Readout"=w453:enum16{"Read Arduino", "Enter manually"}, "Arduino"=w447:refnum<class "ArduinoControl.lvclass">)
      n263 = case shown="\"Read Arduino\"" w453 {
        tunnel: w447 -> [_ w494]
        frame "Enter manually", Default {
        }
        frame "Read Arduino" {
          n264 = call "ArduinoClose.vi"("ArduinoControl in"=w494) -> ()  [unwired: 9 in, 2 out]
        }
      }
      n265 = case shown="True" w455 {
        tunnel: [FALSE w499] -> w457
        frame False {
        }
        frame True {
          n266 = Two Button Dialog(message="Are you sure you don't want to save the data?", 1:"Quit" ("F button name (\"Cancel\")"), 2:"Save data" ("T button name (\"OK\")")) -> (T button?=w499:bool)
        }
      }
      n267 = Or(x=w456, y=w457) -> (x .or. y?=w452:bool)
      n268 = flat-sequence {
        tunnel: w452 -> [w479]
        tunnel: [w479] -> w448
        tunnel: [TRUE] -> w446
        frame #0 {
          w466 = "%010.2f"
          w471 = T3."Read Array" ("Action")
          n269 = local write "STATUS 1"("Saving Data ...") -> ()
          n270 = global read "QC_MeasurementSetup.vi" "Ris Measurement Parameters"() -> (w490:T7)
          n271 = call "RisData.vi"("Action"=w471, "Array No."=u32 1 ("Action")) -> ("Array OUT"=w484:dbl[])  [unwired: 3 in, 1 out]
          n272 = call "RisData.vi"("Action"=w471, "Array No."=u32 2 ("Action")) -> ("Array OUT"=w469:dbl[])  [unwired: 3 in, 1 out]
          n273 = call "RisData.vi"("Action"=w471, "Array No."=u32 0 ("Action")) -> ("Array OUT"=w463:dbl[])  [unwired: 3 in, 1 out]
          n274 = Build Array(w463, w484, w469) -> (w483:dbl[][])
          n275 = call "RisData.vi"("Action"=w471, "Array No."=u32 4 ("Action")) -> ("Array OUT"=w489:dbl[])  [unwired: 3 in, 1 out]
          n276 = call "RisData.vi"("Action"=w471, "Array No."=u32 3 ("Action")) -> ("Array OUT"=w464:dbl[])  [unwired: 3 in, 1 out]
          n277 = Unbundle By Name(w490) -> ("R_is Limit [MOhm]"=w473:dbl, "Number Of Steps"=w460:u32)
          n278 = call <vilib>:"Std Deviation and Variance.vi"("X"=w489) -> ("mean"=w480:dbl)  [unwired: 1 in, 2 out]
          n279 = call <vilib>:"Std Deviation and Variance.vi"("X"=w464) -> ("mean"=w481:dbl)  [unwired: 1 in, 2 out]
          n280 = Transpose 2D Array(2D array=w483) -> (transposed array=w482:dbl[][])
          n281 = local read "Ris induced Voltage [V]"() -> (w467:dbl[][][])
          n282 = local read "Ris SMU Current [nA]"() -> (w468:dbl[][][])
          n283 = call "ScanFeedback.vi"("measurement type"=T1."Ris") -> ("V breakdown"=w475:dbl)  [unwired: 4 in, 4 out]
          n284 = call "SaveDataFile.vi"("Data Array"=w482, "Temperature"=w481, "Humidity"=w480, "no. of arrays"=2, "Actual array lengths"=w460, "Array Titles"="Voltage[V] Current[nA] R_is[MOhm]", "Strip Segment"="", "Arrays format"=w466) -> ("Path + Filename OUT"=w465:string, "Error Out"=w462:errorcluster)  [unwired: 4 in, 2 out]
          n285 = Absolute Value(x=w475) -> (abs(x)=w474:dbl)
          n286 = Absolute Value(x=w473) -> (abs(x)=w472:dbl)
          n287 = call "SaveRisRawData.vi"("Filename"=w465, "Induced Voltage [V]"=w467, "Volts"=w463, "error in (no error)"=w462, "SMU Current [nA]"=w468, "Data formats"=w466, "Number of data points"=w460) -> ("error out"=w461:errorcluster)  [unwired: 3 in]
          n288 = Greater Or Equal?(x=w474, y=w472) -> (x >= y?=w476:bool)
          n289 = call "WriteLogFile.vi"("Automatic warning"="", "Data File"=w465, "Error In"=w461, "DUT passed?"=w476, "Value TechSpec criteria"=w475, "Files saved?"=w479) -> ()  [unwired: 5 in, 1 out]
        }
      }
      n290 = Select(t="Run finished.\nData saved." ("STATUS 1"), s=w448, f="Run finished.\nData not saved." ("STATUS 1")) -> (s? t:f=w451:string)
      n291 = local write "STATUS 1"(w451) -> ()
      "Done!" <- w446
    }
  }
